vi "clearValue.vi"(8 "error in (no error)":errorcluster, 11 "StaticOutputEditor in":refnum<class "StaticOutputEditor.lvclass">) -> (0 "error out":errorcluster, 3 "StaticOutputEditor out":refnum<class "StaticOutputEditor.lvclass">)   [LabVIEW 2011, in "Views.lvlib" / "ScriptEditor.lvlib" / "StaticOutputEditor.lvclass"]
uses:
  StaticOutputEditor.lvclass
  StaticOutputEditor.lvclass/StaticOutputEditor.ctl
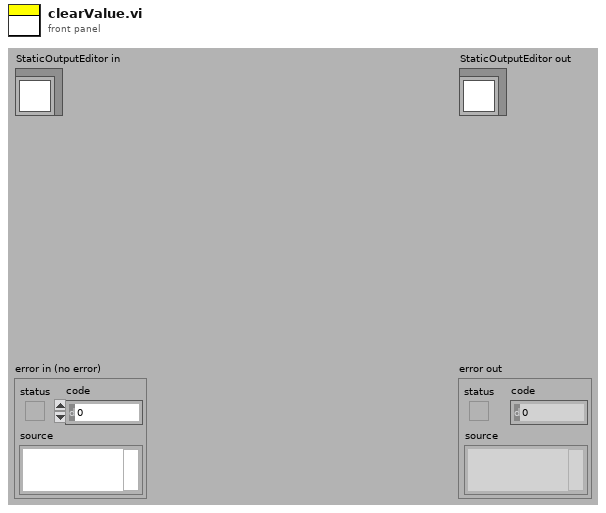
[diagram p1: front panel]
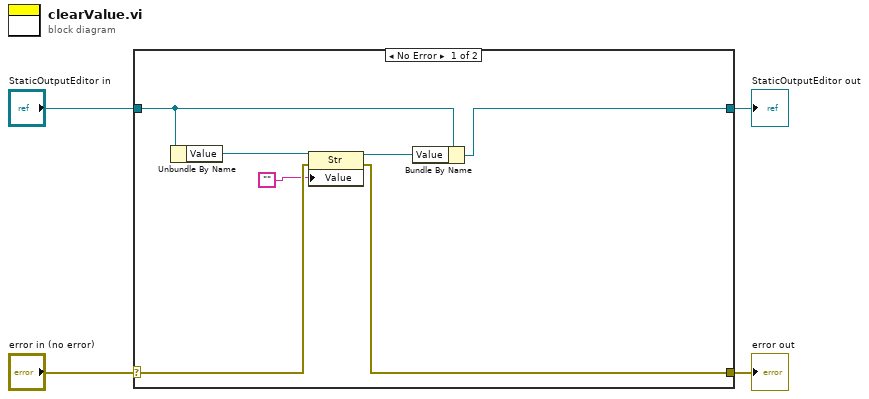
[diagram p0: block diagram]
diagram:
  n1 = case shown="No Error" "error in (no error)" {
    selector: "error in (no error)" -> [w10 w13]
    tunnel: [w8 w13] -> w3
    tunnel: [w5 w12] -> w1
    tunnel: "StaticOutputEditor in" -> [w6 w12]
    frame No Error {
      n2 = Unbundle By Name(w6) -> ("Value"=w11:refnum<vi>)
      n3 = property class="Str"(reference=w11, error in=w10, "Value"="") -> (reference out=w7:refnum<vi>, error out=w8:errorcluster)
      n4 = Bundle By Name(cluster=w6, "Value"=w7) -> (w5:refnum<class "StaticOutputEditor.lvclass">)
    }
    frame Error {
    }
  }
  "error out" <- w3
  "StaticOutputEditor out" <- w1
